vi "V_Rep_demo_Vincent.vi"() -> ()   [LabVIEW 2019]
uses:
  <userlib>/V-REP/V-REP.lvlib
panel:
  in  "operationMode 2":i32
  out "error out 2":errorcluster
  out "error out":errorcluster
  out "function return 2":i32
  out "objectCount out":i32
  in  "stop":bool
  in  "operationMode":i32
  out "function return":i32
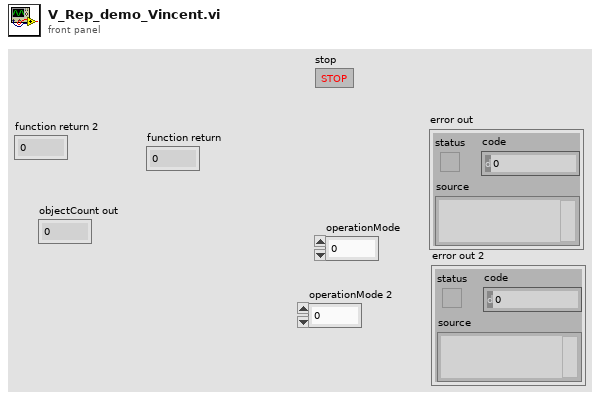
[diagram p1: front panel]
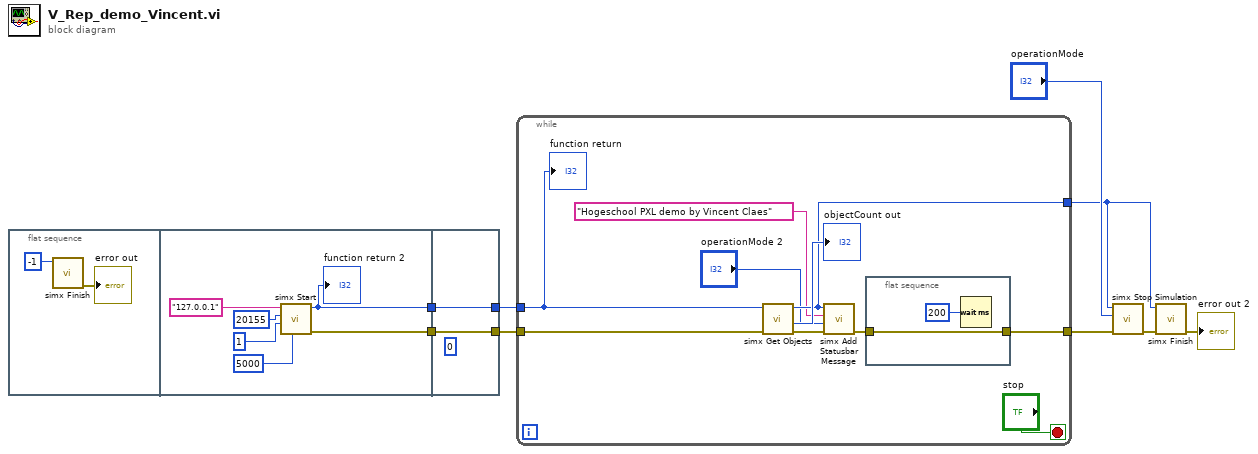
[diagram p0: block diagram]
diagram:
  n1 = flat-sequence {
    tunnel: [w14] -> w5
    tunnel: [w13] -> w4
    tunnel: [w19] -> w6
    tunnel: [w18] -> w7
    tunnel: w5 -> [w18]
    tunnel: w4 -> [w19]
    frame #0 {
      n2 = call <userlib>:"simx Finish.vi"("clientID"=-1) -> ("error out"=→"error out":errorcluster)  [unwired: 10 in]
    }
    frame #1 {
      n3 = call <userlib>:"simx Start.vi"("timeOutInMs"=5000, "waitUntilConnected"=u8 1, "connectionPort"=20155, "connectionAddress"="127.0.0.1") -> ("error out"=w14:errorcluster, "function return"=w13:i32)  [unwired: 6 in]
      "function return 2" <- w13
    }
    frame #2 {
      (unwired) 0 ("operationMode")
    }
  }
  n4 = while {
    tunnel: w6 -> [w21]
    tunnel: w7 -> [w27]
    tunnel: [w26] -> w8
    tunnel: [w25] -> w3
    stop <- "stop" stop-if-true
    n5 = call <userlib>:"simx Get Objects.vi"("error in (no error)"=w27, "clientID"=w21) -> ("error out"=w23:errorcluster, "objectCount out"=→"objectCount out":i32, "function return"=w25:i32)  [unwired: 6 in, 1 out]
    n6 = call <userlib>:"simx Add Statusbar Message.vi"("error in (no error)"=w23, "operationMode"="operationMode 2", "message"="Hogeschool PXL demo by Vincent Claes", "clientID"=w25) -> ("error out"=w22:errorcluster)  [unwired: 6 in, 1 out]
    n7 = flat-sequence {
      tunnel: w22 -> [w30]
      tunnel: [w30] -> w26
      frame #0 {
        n8 = Wait (ms)(milliseconds to wait=u32 200) -> ()  [unwired: 1 out]
      }
    }
    "function return" <- w21
  }
  n9 = call <userlib>:"simx Stop Simulation.vi"("error in (no error)"=w8, "operationMode"="operationMode", "clientID"=w3) -> ("error out"=w2:errorcluster)  [unwired: 7 in, 1 out]
  n10 = call <userlib>:"simx Finish.vi"("error in (no error)"=w2, "clientID"=w3) -> ("error out"=→"error out 2":errorcluster)  [unwired: 9 in]
